vi "MU Calibration Number Of Nonius Curve Samples.vi"(8 "error in (no error)":errorcluster, 11 "CalibrationAnalyzeResult":T1) -> (0 "error out":errorcluster, 3 "NumberOfNoniusCurveSamples":u64)   [LabVIEW 2017, in "MU_3SL_interface.lvlib"]
uses:
  MU_3SL_interface.lvlib
  handles/CalibrationAnalyzeResultHandle.ctl
  lib/MU_3SL_interface.dll
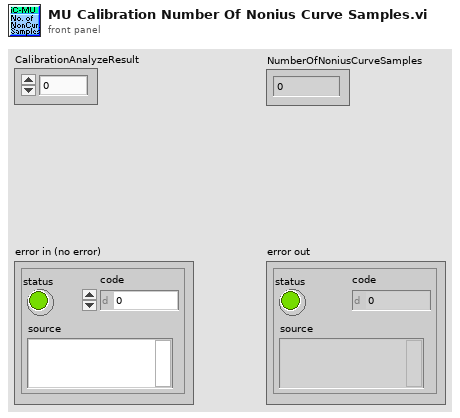
[diagram p1: front panel]
types:
  T1 = typedef "MU_3SL_interface.lvlib/CalibrationAnalyzeResultHandle.ctl" = u64
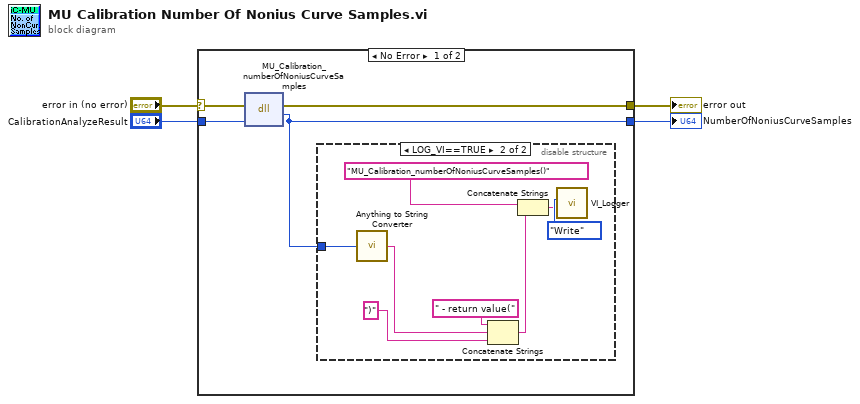
[diagram p0: block diagram]
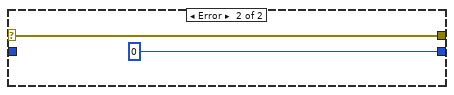
[diagram p3: hidden frame]
diagram:
  n1 = case shown="No Error" "error in (no error)" {
    selector: "error in (no error)" -> [w6 w18]
    tunnel: "CalibrationAnalyzeResult" -> [w8 _]
    tunnel: [w7 w18] -> w4
    tunnel: [w5 u64 0 ("return type")] -> w3
    frame No Error {
      n2 = dll-call lib="C:/Users/bes/AppData/Roaming/work/mu_9so/icsubmodules/soft_mu_3sl_master/lv_interface/lib/MU_3SL_interface**.*" fn="MU_Calibration_numberOfNoniusCurveSamples"(error in=w6, "analyzeResult"=w8) -> (error out=w7:errorcluster, "NumberOfNoniusPhaseErrorSamples"=w5:u64)  [unwired: 3 in, 1 out]
      n3 = disable-structure shown="LOG_VI==TRUE" {
        disable-tunnel: w5 -> [_ w10]
        frame condition #0 {
        }
        frame condition #1 (active) {
          n4 = call "Anything to String Converter.vi"("anything"=w10) -> ("String"=w9:string)
          n5 = Concatenate Strings(" - return value(" ("string"), w9, ")" ("string")) -> (w14:string)
          n6 = Concatenate Strings("MU_Calibration_numberOfNoniusCurveSamples()" ("Info in"), w14) -> (w13:string)
          n7 = call "VI_Logger.vi"("Action (Read)"=enum16{"Write", "Read"}."Write", "Info in"=w13) -> ()  [unwired: 8 in, 2 out]
        }
      }
    }
    frame Error {
    }
  }
  "error out" <- w4
  "NumberOfNoniusCurveSamples" <- w3
